vi "Generate Python.vi"(8 "error in (no error)":errorcluster, 11 "PyTool in":refnum<class "PyTool.lvclass">) -> (0 "error out":errorcluster, 2 "Python Code":string, 3 "PyTool out":refnum<class "PyTool.lvclass">)   [LabVIEW 2025, in "Tools.lvlib" / "PyTool.lvclass"]
uses:
  PyTool.lvclass
  PyTool.lvclass/PyTool.ctl
  Tools.lvlib
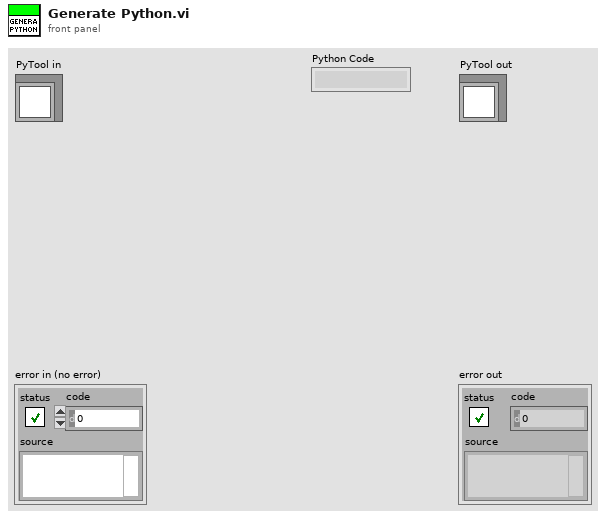
[diagram p1: front panel]
types:
  T1 = typedef "Tools.lvlib/PyTool.lvclass/Parameter.ctl" = cluster{"Name":string, "type":T2, "Input?":bool, "Ignored?":bool, "Exception Value":string, "Description":string}
  T2 = typedef "Tools.lvlib/Datatypes.ctl" = enum16{"Float", "Int", "String", "String Array", "Int Array", "Float Array", "Bool Array", "Bool", "Invalid"}
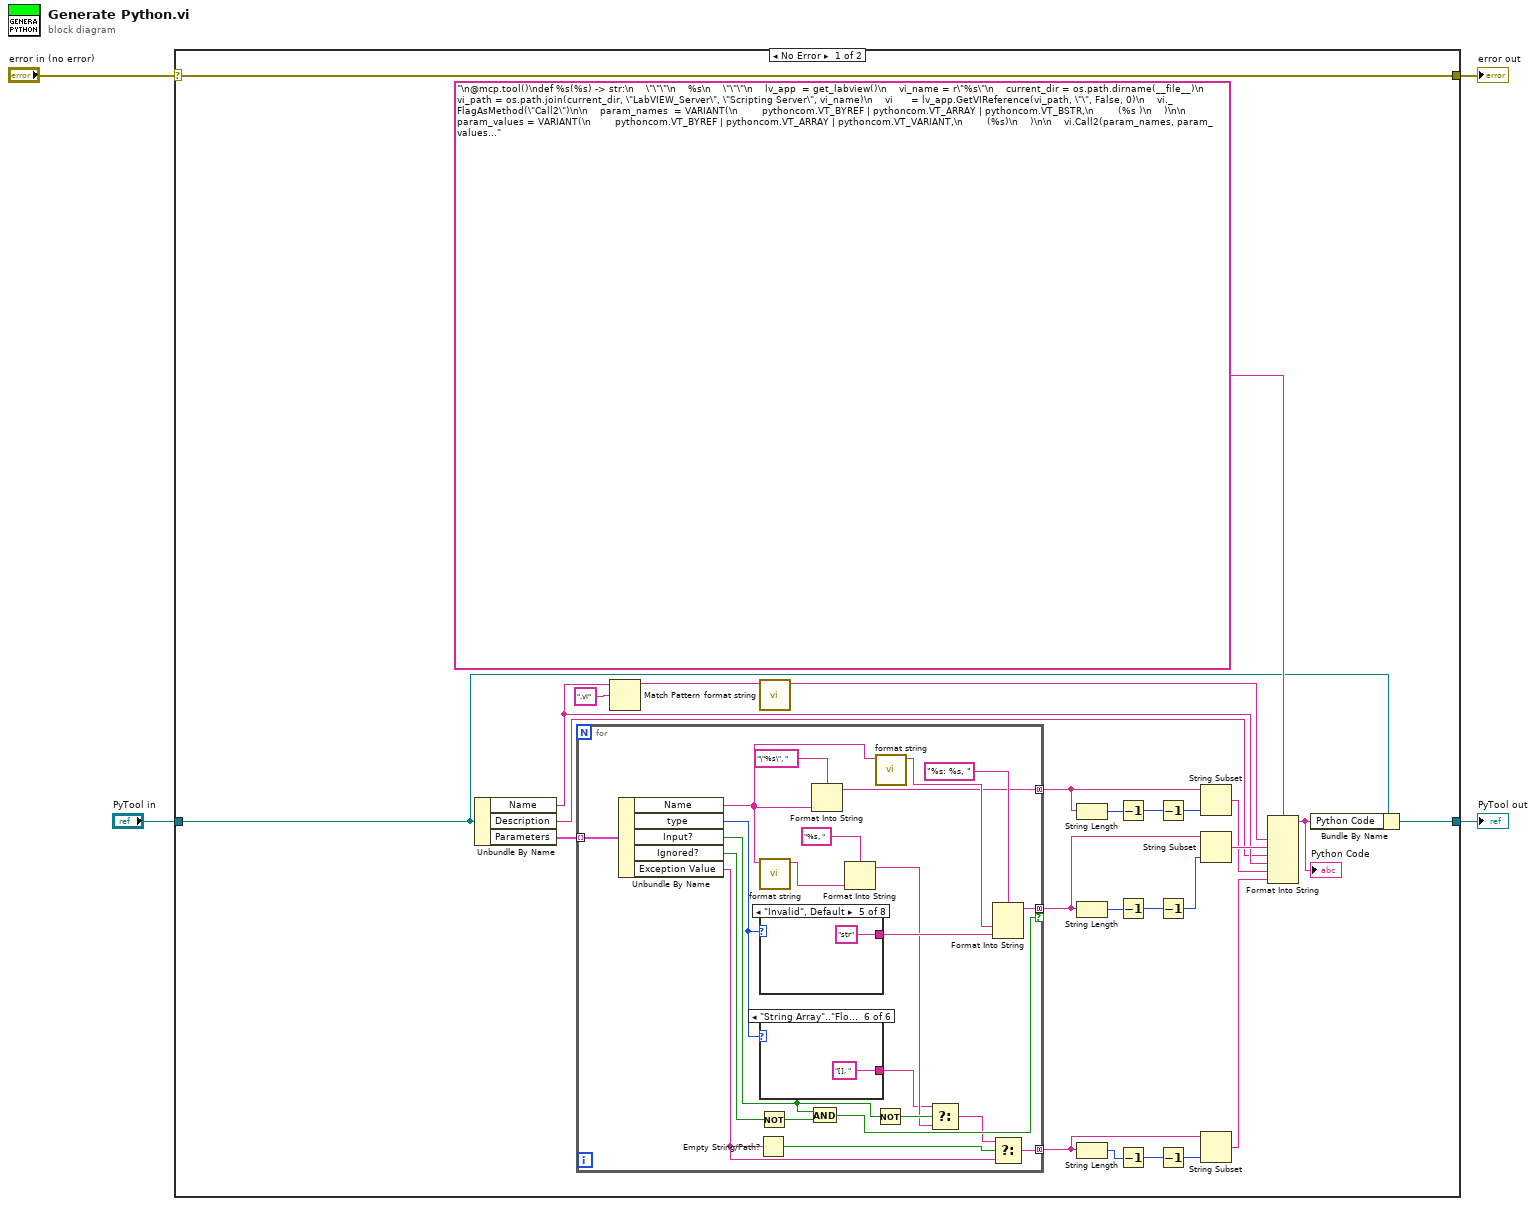
[diagram p0: block diagram]
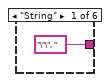
[diagram p2: hidden frame]
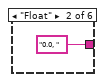
[diagram p3: hidden frame]
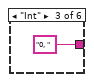
[diagram p4: hidden frame]
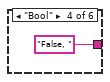
[diagram p5: hidden frame]
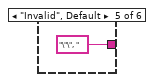
[diagram p6: hidden frame]
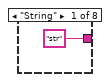
[diagram p7: hidden frame]
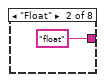
[diagram p8: hidden frame]
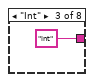
[diagram p9: hidden frame]
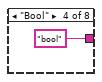
[diagram p10: hidden frame]
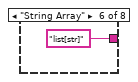
[diagram p11: hidden frame]
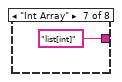
[diagram p12: hidden frame]
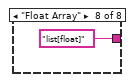
[diagram p13: hidden frame]
diagram:
  n1 = case shown="No Error" "error in (no error)" {
    selector: "error in (no error)" -> [w30 w68]
    tunnel: [w30 w68] -> w3
    tunnel: [w6 w67] -> w1
    tunnel: "PyTool in" -> [w12 w67]
    frame No Error {
      n2 = Unbundle By Name(w12) -> ("Name"=w11:string, "Description"=w10:string, "Parameters"=w9:T1[])
      n3 = for {
        tunnel: [w50] -> w23 mode=concatenating if=w49
        tunnel: w9 -> [w46] mode=indexing
        tunnel: [w44] -> w8 mode=concatenating
        tunnel: [w32] -> w7 mode=concatenating
        n4 = Unbundle By Name(w46) -> ("Name"=w36:string, "type"=w35:T2, "Input?"=w34:bool, "Ignored?"=w33:bool, "Exception Value"=w31:string)
        n5 = Empty String/Path?(string/path=w31) -> (empty?=w43:bool)
        n6 = Not(x=w33) -> (.not. x?=w48:bool)
        n7 = call "format string.vi"("Label.Text"=w36) -> ("String"=w39:string)  [unwired: 10 in]
        n8 = case shown="\"Invalid\", Default" w35 {
          tunnel: ["str" ("format string") "float" ("format string") "int" ("format string") "bool" ("format string") "str" ("format string") "list[str]" ("format string") "list[int]" ("format string") "list[float]" ("format string")] -> w51
          frame "String" {
          }
          frame "Float" {
          }
          frame "Int" {
          }
          frame "Bool" {
          }
          frame "Invalid", Default {
          }
          frame "String Array" {
          }
          frame "Int Array" {
          }
          frame "Float Array" {
          }
        }
        n9 = case shown="\"String Array\"..\"Float Array\"" w35 {
          tunnel: ["\"\", " ("format string") "0.0, " ("format string") "0, " ("format string") "False, " ("format string") "\"\", " ("format string") "[], " ("format string")] -> w38
          frame "String" {
          }
          frame "Float" {
          }
          frame "Int" {
          }
          frame "Bool" {
          }
          frame "Invalid", Default {
          }
          frame "String Array".."Float Array" {
          }
        }
        n10 = And(x=w34, y=w48) -> (x .and. y?=w49:bool)
        n11 = Format Into String(format string="\"%s\", ", w36) -> (resulting string=w44:string)  [unwired: 2 in, 1 out]
        n12 = Format Into String(format string="%s, ", w39) -> (resulting string=w41:string)  [unwired: 2 in, 1 out]
        n13 = Not(x=w34) -> (.not. x?=w42:bool)
        n14 = call "format string.vi"("Label.Text"=w36) -> ("String"=w47:string)  [unwired: 10 in]
        n15 = Select(t=w38, s=w42, f=w41) -> (s? t:f=w37:string)
        n16 = Format Into String(format string="%s: %s, ", w47, w51) -> (resulting string=w50:string)  [unwired: 2 in, 1 out]
        n17 = Select(t=w37, s=w43, f=w31) -> (s? t:f=w32:string)
      }
      n18 = Match Pattern(string=w11, regular expression=".vi") -> (before substring=w28:string)  [unwired: 1 in, 3 out]
      n19 = call "format string.vi"("Label.Text"=w28) -> ("String"=w21:string)  [unwired: 10 in]
      n20 = String Length(string=w8) -> (length=w19:i32)
      n21 = String Length(string=w23) -> (length=w25:i32)
      n22 = String Length(string=w7) -> (length=w15:i32)
      n23 = Decrement(x=w19) -> (x-1=w18:i32)
      n24 = Decrement(x=w25) -> (x-1=w24:i32)
      n25 = Decrement(x=w15) -> (x-1=w16:i32)
      n26 = Decrement(x=w18) -> (x-1=w20:i32)
      n27 = Decrement(x=w24) -> (x-1=w26:i32)
      n28 = Decrement(x=w16) -> (x-1=w14:i32)
      n29 = String Subset(string=w8, length (rest)=w20) -> (substring=w17:string)  [unwired: 1 in]
      n30 = String Subset(string=w23, length (rest)=w26) -> (substring=w22:string)  [unwired: 1 in]
      n31 = String Subset(string=w7, length (rest)=w14) -> (substring=w13:string)  [unwired: 1 in]
      n32 = Format Into String(format string="\n@mcp.tool()\ndef %s(%s) -> str:\n    \"\"\"\n    %s\n    \"\"\"\n    lv_app  = get_labview()\n    vi_name = r\"%s\"\n    current_dir = os.path.dirname(__file__)\n    vi_path = os.path.join(current_dir, \"LabVIEW_Server\", \"Scripting Server\", vi_name)\n    vi      = lv_app.GetVIReference(vi_path, \"\", False, 0)\n    vi._FlagAsMethod(\"Call2\")\n\n    param_names  = VARIANT(\n        pythoncom.VT_BYREF | pythoncom.VT_ARRAY | pythoncom.VT_BSTR,\n        (%s )\n    )\n\n    param_values = VARIANT(\n        pythoncom.VT_BYREF | pythoncom.VT_ARRAY | pythoncom.VT_VARIANT,\n        (%s)\n    )\n\n    vi.Call2(param_names, param_values,\n            False,   # open FP?\n            False,   # close FP after call?\n            False,   # suspend on call?\n            False)   # bring LabVIEW to front?\n    \n    return param_values\n\n", w21, w22, w10, w11, w17, w13) -> (resulting string=w5:string)  [unwired: 2 in, 1 out]
      "Python Code" <- w5
      n33 = Bundle By Name(cluster=w12, "Python Code"=w5) -> (w6:refnum<class "PyTool.lvclass">)
    }
    frame Error {
    }
  }
  "error out" <- w3
  "PyTool out" <- w1
